vi "TL27_Get_Single_Fault_Snapshot.vi"(0 "GEA2 Reference In":refnum<k24>, 5 "Standalone?":bool, 7 "Snapshot Selection":T2, 11 "Error In":errorcluster) -> (4 "GEA2 Reference Out":refnum<k24>, 6 "Fault Snapshots":T1, 15 "Error Out":errorcluster)   [LabVIEW 2021]
uses:
  subVIs/Snap_Selection.ctl
  D:/Common/LabVIEW GEA2 Toolkit/source/GEA3 DLL Source/GeaCommunication.dll
  Common/LabVIEW GEA2 Toolkit/source/GEA3 DLL Source/GeaCommunication.dll
  subVIs/Snap_Input.ctl
  Common/LabVIEW GEA2 Toolkit/GEA3/type defs/Source_Destination.ctl
  Common/LabVIEW GEA2 Toolkit/GEA3/type defs/ERD Read Data In.ctl
  Common/LabVIEW GEA2 Toolkit/GEA3/library/GEA2_Toolkit.lvlib
panel:
  out "ERD Number":string
  out "ERD Data":string
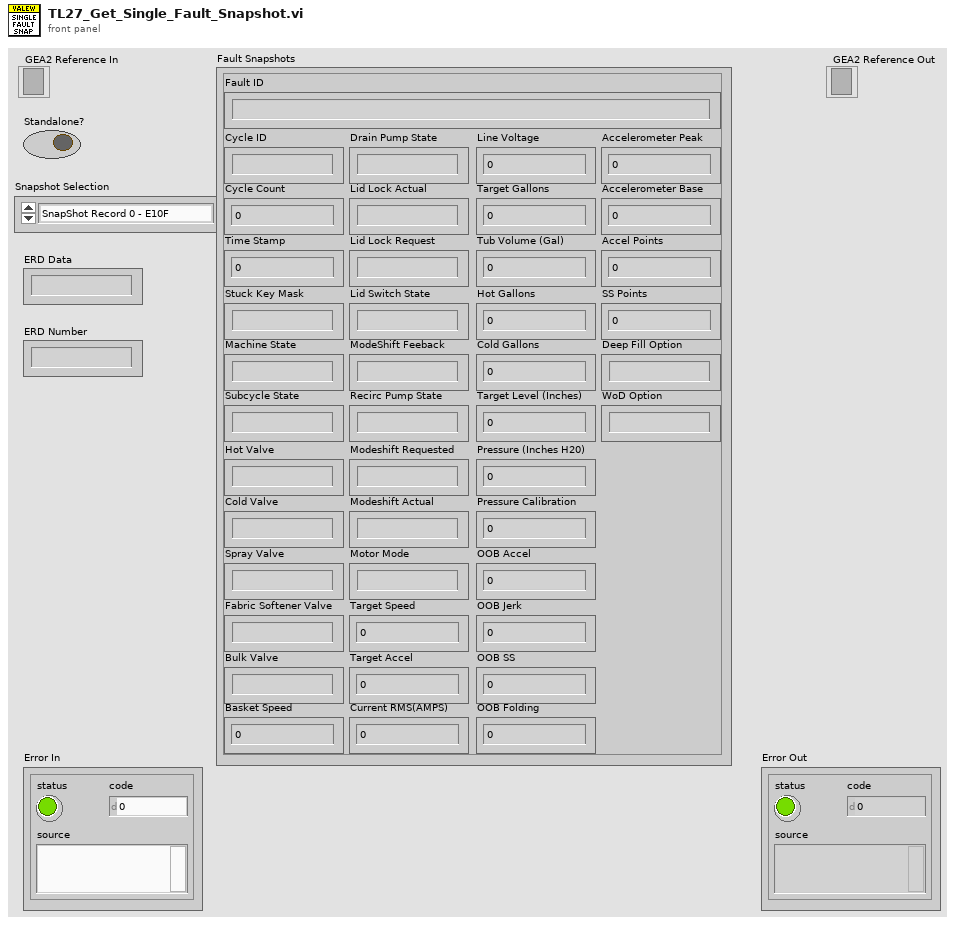
[diagram p1: front panel]
types:
  T1 = typedef "Snap_Input.ctl" = cluster{"Fault ID":string, "Cycle Count":u32, "Cycle ID":string, "Time Stamp":u32, "Stuck Key Mask":string, "Machine State":string, "Subcycle State":string, "Hot Valve":string, "Cold Valve":string, "Spray Valve":string, "Fabric Softener Valve":string, "Bulk Valve":string, "Drain Pump State":string, "Lid Lock Actual":string, "Lid Lock Request":string, "Lid Switch State":string, "ModeShift Feeback":string, "Recirc Pump State":string, "Modeshift Requested":string, "Modeshift Actual":string, "Motor Mode":string, "Target Speed":u16, "Target Accel":u16, "Current RMS(AMPS)":dbl, "Line Voltage":dbl, "Target Gallons":dbl, "Tub Volume (Gal)":dbl, "Hot Gallons":dbl, "Cold Gallons":dbl, "Target Level (Inches)":dbl, "Pressure (Inches H20) ":dbl, "Pressure Calibration":dbl, "OOB Accel":i32, "OOB Jerk":i32, "OOB SS":i32, "OOB Folding":i32, "Accelerometer Peak":i16, "Accelerometer Base":i16, "Accel Points":u8, "SS Points":u8, "Deep Fill Option":string, "WoD Option":string, "Basket Speed":u16}
  T2 = typedef "Snap_Selection.ctl" = enum16{"SnapShot Record 0 - E10F", "Snapshot Record 1 - E110", "Snapshot Record 2 - E111", "Snapshot Record 3 - E112", "Snapshot Record 4 - E113", "Snapshot Record 5 - E114", "Snapshot Record 6 - E115", "Snapshot Record 7 - E116", "Snapshot Record 8 - E117", "Snapshot Record 9 - E118"}
  T3 = typedef "Source_Destination.ctl" = cluster{"Source":u8, "Destination":u8}
  T4 = typedef "ERD Read Data In.ctl" = cluster{"ERD Number":u16, "Data Type":enum16{"string", "boolean", "uint8_t", "uint16_t", "uint32_t", "uint64_t", "int8_t", "int16_t", "int32_t", "int64_t"}}
  T5 = typedef "ERD Read Data Out.ctl" = cluster{"ERD Number":u16, "Data":string}
  T6 = cluster{"ERD Data Out[0]":T5, "ERD Data Out[1]":T5, "ERD Data Out[2]":T5, "ERD Data Out[3]":T5, "ERD Data Out[4]":T5, "ERD Data Out[5]":T5, "ERD Data Out[6]":T5, "ERD Data Out[7]":T5, "ERD Data Out[8]":T5}
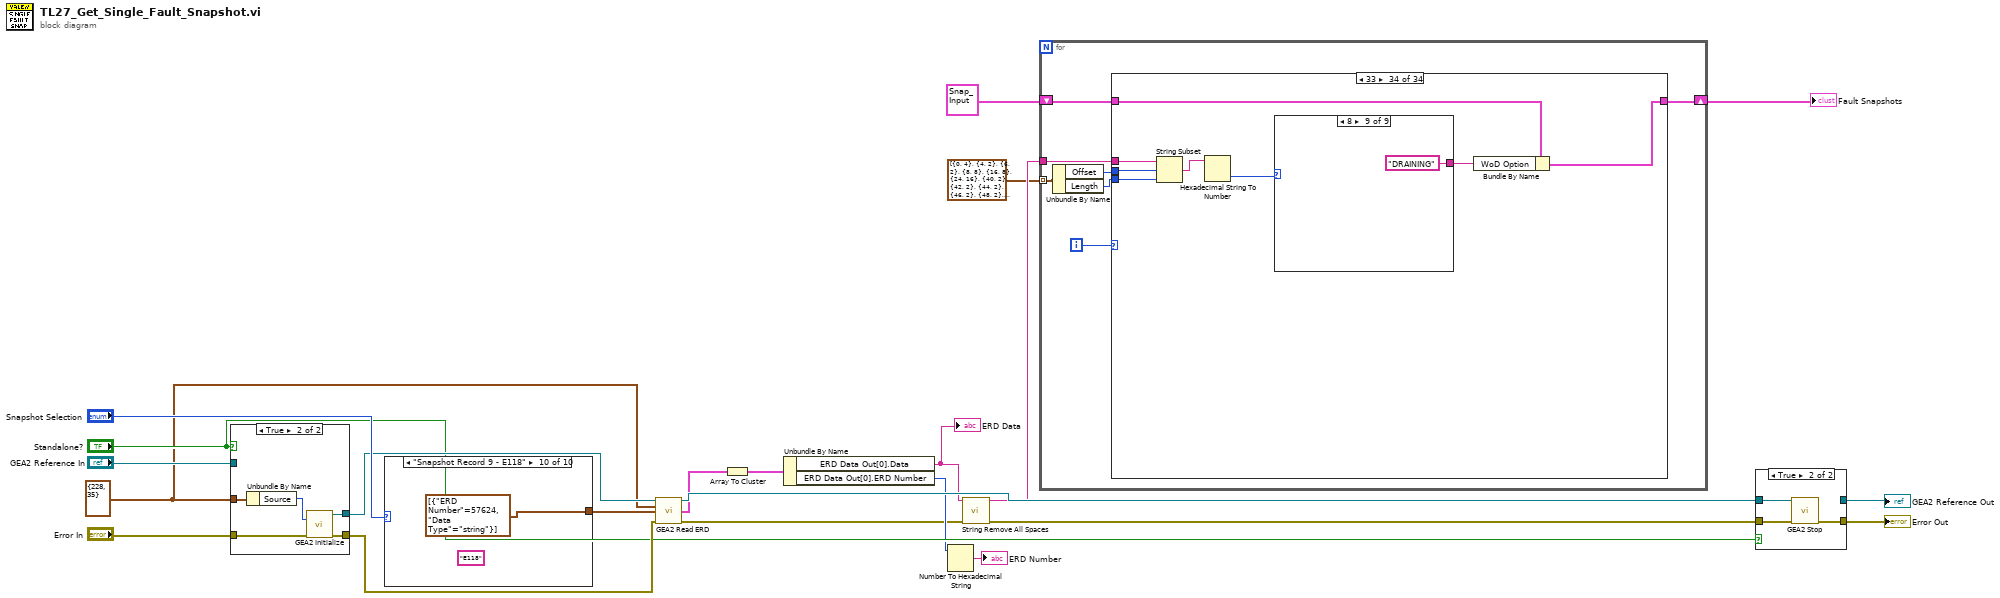
[diagram p0: block diagram]
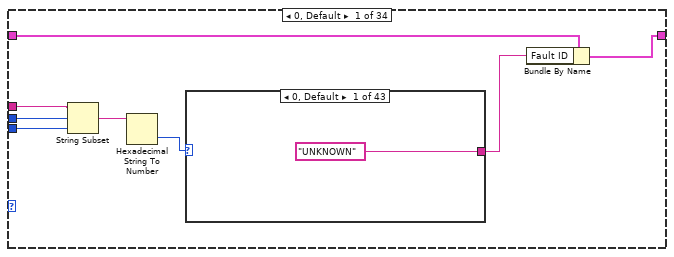
[diagram p2: hidden frame]
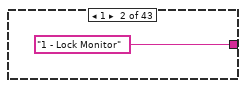
[diagram p3: hidden frame]
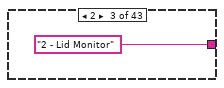
[diagram p4: hidden frame]
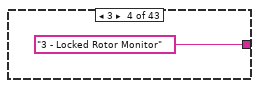
[diagram p5: hidden frame]
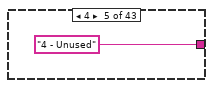
[diagram p6: hidden frame]
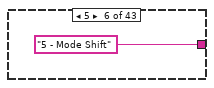
[diagram p7: hidden frame]
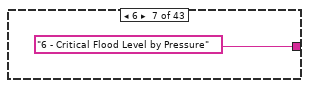
[diagram p8: hidden frame]
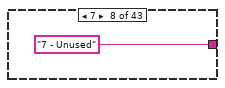
[diagram p9: hidden frame]
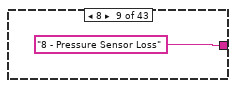
[diagram p10: hidden frame]
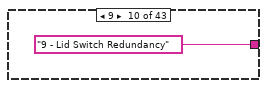
[diagram p11: hidden frame]
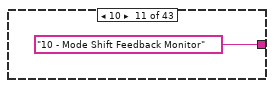
[diagram p12: hidden frame]
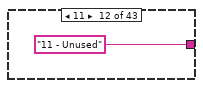
[diagram p13: hidden frame]
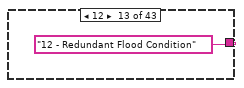
[diagram p14: hidden frame]
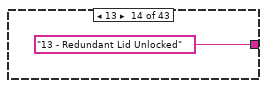
[diagram p15: hidden frame]
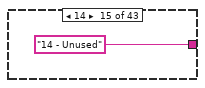
[diagram p16: hidden frame]
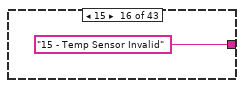
[diagram p17: hidden frame]
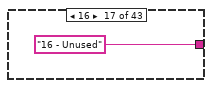
[diagram p18: hidden frame]
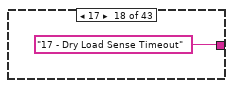
[diagram p19: hidden frame]
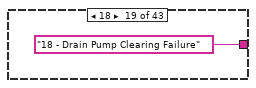
[diagram p20: hidden frame]
diagram:
  w13 = T3 {"Source"=228, "Destination"=35} ("GEA Inputs")
  n1 = case shown="True" "Standalone?" {
    tunnel: "Error In" -> [w23 w29]
    tunnel: [w23 w28] -> w17
    tunnel: "GEA2 Reference In" -> [w24 _]
    tunnel: [w24 w27] -> w18
    tunnel: w13 -> [_ w25]
    frame False {
    }
    frame True {
      n2 = Unbundle By Name(w25) -> ("Source"=w26:u8)
      n3 = call "GEA2 Initialize.vi"("Source Address"=w26, "error in"=w29) -> ("GEA2 Reference Out"=w27:refnum<k24>, "error out"=w28:errorcluster)  [unwired: 10 in, 2 out]
    }
  }
  n4 = case shown="\"Snapshot Record 9 - E118\"" "Snapshot Selection" {
    tunnel: [T4[] [{"ERD Number"=57615, "Data Type"=enum."string"}] ("Read ERD List") T4[] [{"ERD Number"=57616, "Data Type"=enum."string"}] ("Read ERD List") T4[] [{"ERD Number"=57617, "Data Type"=enum."string"}] ("Read ERD List") T4[] [{"ERD Number"=57618, "Data Type"=enum."string"}] ("Read ERD List") T4[] [{"ERD Number"=57619, "Data Type"=enum."string"}] ("Read ERD List") T4[] [{"ERD Number"=57620, "Data Type"=enum."string"}] ("Read ERD List") T4[] [{"ERD Number"=57621, "Data Type"=enum."string"}] ("Read ERD List") T4[] [{"ERD Number"=57622, "Data Type"=enum."string"}] ("Read ERD List") T4[] [{"ERD Number"=57623, "Data Type"=enum."string"}] ("Read ERD List") T4[] [{"ERD Number"=57624, "Data Type"=enum."string"}] ("Read ERD List")] -> w21
    frame "SnapShot Record 0 - E10F", Default {
      (unwired) "E10F"
    }
    frame "Snapshot Record 1 - E110" {
      (unwired) "E110"
    }
    frame "Snapshot Record 2 - E111" {
      (unwired) "E111"
    }
    frame "Snapshot Record 3 - E112" {
      (unwired) "E112"
    }
    frame "Snapshot Record 4 - E113" {
      (unwired) "E113"
    }
    frame "Snapshot Record 5 - E114" {
      (unwired) "E114"
    }
    frame "Snapshot Record 6 - E115" {
      (unwired) "E115"
    }
    frame "Snapshot Record 7 - E116" {
      (unwired) "E116"
    }
    frame "Snapshot Record 8 - E117" {
      (unwired) "E117"
    }
    frame "Snapshot Record 9 - E118" {
      (unwired) "E118"
    }
  }
  n5 = call "GEA2 Read ERD.vi"("GEA2 Reference In"=w18, "GEA Inputs"=w13, "Read ERD List"=w21, "Error In"=w17) -> ("GEA2 Reference Out"=w16:refnum<k24>, "ERD Data Out"=w12:T5[], "Error Out"=w7:errorcluster)  [unwired: 8 in, 1 out]
  n6 = Array To Cluster(array=w12) -> (cluster=w11:T6)
  n7 = Unbundle By Name(w11) -> ("ERD Data Out[0].Data"=w8:string, "ERD Data Out[0].ERD Number"=w10:u16)
  "ERD Data" <- w8
  n8 = Number To Hexadecimal String(2:w10) -> (0:→"ERD Number":string)  [unwired: 1 in]
  n9 = call "String Remove All Spaces.vi"("Input String"=w8, "error in (no error)"=w7) -> ("Spaces Removed"=w4:string, "error out"=w6:errorcluster)  [unwired: 12 in]
  n10 = for {
    tunnel: w4 -> [w46]
    shift-right: [w44] -> w1
    shift-left: T1 {"Fault ID"="", "Cycle Count"=0, "Cycle ID"="", "Time Stamp"=0, "Stuck Key Mask"="", "Machine State"="", "Subcycle State"="", "Hot Valve"="", "Cold Valve"="", "Spray Valve"="", "Fabric Softener Valve"="", "Bulk Valve"="", "Drain Pump State"="", "Lid Lock Actual"="", "Lid Lock Request"="", "Lid Switch State"="", "ModeShift Feeback"="", "Recirc Pump State"="", "Modeshift Requested"="", "Modeshift Actual"="", "Motor Mode"="", "Target Speed"=0, "Target Accel"=0, "Current RMS(AMPS)"=0.0, "Line Voltage"=0.0, "Target Gallons"=0.0, "Tub Volume (Gal)"=0.0, "Hot Gallons"=0.0, "Cold Gallons"=0.0, "Target Level (Inches)"=0.0, "Pressure (Inches H20) "=0.0, "Pressure Calibration"=0.0, "OOB Accel"=0, "OOB Jerk"=0, "OOB SS"=0, "OOB Folding"=0, "Accelerometer Peak"=0, "Accelerometer Base"=0, "Accel Points"=0, "SS Points"=0, "Deep Fill Option"="", "WoD Option"="", "Basket Speed"=0} ("input cluster") -> [w45]
    tunnel: cluster{"Offset":i32, "Length":i32}[] [{"Offset"=0, "Length"=4}, {"Offset"=4, "Length"=2}, {"Offset"=6, "Length"=2}, {"Offset"=8, "Length"=8}, {"Offset"=16, "Length"=8}, {"Offset"=24, "Length"=16}, {"Offset"=40, "Length"=2}, {"Offset"=42, "Length"=2}, {"Offset"=44, "Length"=2}, {"Offset"=46, "Length"=2}, {"Offset"=48, "Length"=2}, {"Offset"=50, "Length"=2}, {"Offset"=52, "Length"=4}, {"Offset"=56, "Length"=4}, {"Offset"=60, "Length"=4}, {"Offset"=64, "Length"=4}, {"Offset"=68, "Length"=4}, {"Offset"=72, "Length"=4}, {"Offset"=76, "Length"=4}, {"Offset"=80, "Length"=4}, {"Offset"=84, "Length"=4}, {"Offset"=88, "Length"=8}, {"Offset"=96, "Length"=8}, {"Offset"=104, "Length"=8}, {"Offset"=112, "Length"=8}, {"Offset"=120, "Length"=8}, {"Offset"=128, "Length"=8}, {"Offset"=136, "Length"=8}, {"Offset"=144, "Length"=4}, {"Offset"=148, "Length"=4}, {"Offset"=152, "Length"=2}, {"Offset"=154, "Length"=2}, {"Offset"=156, "Length"=2}, {"Offset"=158, "Length"=2}] -> [w41] mode=indexing
    i -> [w43]
    n11 = Unbundle By Name(w41) -> ("Offset"=w42:i32, "Length"=w40:i32)
    n12 = case shown="33" w43 {
      tunnel: w46 -> [w53 w105 _ w150 w159 w165 w188 w208 w235 w271 w294 w307 w322 w330 w338 w348 w358 w368 w378 w388 w398 w408 w418 w428 w436 w444 w452 w460 w468 w476 w484 w492 w502 w511]
      tunnel: w42 -> [w52 w104 _ w149 w158 w164 w187 w207 w234 w270 w293 w306 w321 w329 w337 w347 w357 w367 w377 w387 w397 w407 w417 w427 w435 w443 w451 w459 w467 w475 w483 w491 w501 w510]
      tunnel: w40 -> [w51 w103 _ w148 w157 w163 w186 w206 w233 w269 w292 w305 w320 w328 w336 w346 w356 w366 w376 w386 w396 w406 w416 w426 w434 w442 w450 w458 w466 w474 w482 w490 w500 w509]
      tunnel: w45 -> [w54 w102 w145 w152 w156 w167 w190 w205 w237 w273 w296 w309 w324 w332 w340 w350 w360 w370 w380 w390 w400 w410 w420 w430 w438 w446 w454 w462 w470 w478 w486 w494 w499 w513]
      tunnel: [w50 w101 w145 w151 w155 w166 w189 w204 w236 w272 w295 w308 w323 w331 w339 w349 w359 w369 w379 w389 w399 w409 w419 w429 w437 w445 w453 w461 w469 w477 w485 w493 w498 w512] -> w44
      frame 0, Default {
        n13 = String Subset(string=w53, offset (0)=w52, length (rest)=w51) -> (substring=w49:string)
        n14 = Hexadecimal String To Number(string=w49) -> (number=w48:u32)  [unwired: 2 in, 1 out]
        n15 = case shown="0, Default" w48 {
          tunnel: ["UNKNOWN" "1 - Lock Monitor" "2 - Lid Monitor" "3 - Locked Rotor Monitor" "4 - Unused" "5 - Mode Shift" "6 - Critical Flood Level by Pressure" "7 - Unused" "8 - Pressure Sensor Loss" "9 - Lid Switch Redundancy" "10 - Mode Shift Feedback Monitor" "11 - Unused" "12 - Redundant Flood Condition" "13 - Redundant Lid Unlocked" "14 - Unused" "15 - Temp Sensor Invalid" "16 - Unused" "17 - Dry Load Sense Timeout" "18 - Drain Pump Clearing Failure" "19 - UI State Timeout" "20 - Critical Flood Level by Gallons" "21 - Unused " "22 - OOB during dry load sense" "23 - Critical Lid Lock Failure: Can't Lock" "24 - Lid Logic Failure" "25 - Pressure Sensor Dropout" "26 - OOB Redistribution" "27 - Water Accessibility" "28 - ADC Knob Feedback Invalid" "29 - Suds Lock Abatement Failure" "30 - Stuck Button Fault" "31 - OOB Fallback In Final Spin" "32 - Critical Lid Lock Failure: Can't Unlock" "100 - Accelerometer Communication Error" "101 - Max Fill Pressure" "102 - Clock Monitor" "103 - LidLock Failure" "104 - Adaptive Drain" "105 - Max Fill Volume" "106 - Target Spin Speed Timeout" "107 - Target Spin Speed Dropout" "108 - UI-MC Heartbeat Communication Failure" "109 - Event Sequence Buffer Overrun"] -> w47
          frame 0, Default {
          }
          frame 1 {
          }
          frame 2 {
          }
          frame 3 {
          }
          frame 4 {
          }
          frame 5 {
          }
          frame 6 {
          }
          frame 7 {
          }
          frame 8 {
          }
          frame 9 {
          }
          frame 10 {
          }
          frame 11 {
          }
          frame 12 {
          }
          frame 13 {
          }
          frame 14 {
          }
          frame 15 {
          }
          frame 16 {
          }
          frame 17 {
          }
          frame 18 {
          }
          frame 19 {
          }
          frame 20 {
          }
          frame 21 {
          }
          frame 22 {
          }
          frame 23 {
          }
          frame 24 {
          }
          frame 25 {
          }
          frame 26 {
          }
          frame 27 {
          }
          frame 28 {
          }
          frame 29 {
          }
          frame 30 {
          }
          frame 31 {
          }
          frame 32 {
          }
          frame 100 {
          }
          frame 101 {
          }
          frame 102 {
          }
          frame 103 {
          }
          frame 104 {
          }
          frame 105 {
          }
          frame 106 {
          }
          frame 107 {
          }
          frame 108 {
          }
          frame 109 {
          }
        }
        n16 = Bundle By Name(cluster=w54, "Fault ID"=w47) -> (w50:T1)
      }
      frame 1 {
        n17 = String Subset(string=w105, offset (0)=w104, length (rest)=w103) -> (substring=w100:string)
        n18 = Hexadecimal String To Number(string=w100) -> (number=w99:u32)  [unwired: 2 in, 1 out]
        n19 = case shown="0, Default" w99 {
          tunnel: ["0 - NotDefined" "1 - BasketClean" "2 - DrainAndSpin" "3 - QuickRinse" "4 - BulkyItems" "5 - Sanitize" "6 - TowelsSheets" "8 - Normal_Mixedload" "9 - Whites" "10 - DarkColors" "11 - Jeans" "12 - HandWash" "13 - Delicates" "14 - SpeedWash" "15 - HeavyDuty" "16 - Allergen" "17 - PowerClean" "18 - RinseSpin" "19 - SingleItemWash" "20 - Colors" "21 - ColdWash" "22 - WaterOnDemand" "23 - NotUsed_Start" "127 - NotUsed_End" "128 - Cottons" "129 - EasyCare" "130 - ActiveWear" "131 - TimedDry" "132 - DeWrinkle" "133 - QuickAirFluff" "134 - SteamRefresh" "135 - SteamDewrinkle" "136 - SpeedDry" "137 - Mixed" "138 - Quickdry" "139 - Casuals" "140 - Warmup" "141 - EnergySaver" "142 - Antibacterial"] -> w98
          frame 0, Default {
          }
          frame 1 {
          }
          frame 2 {
          }
          frame 3 {
          }
          frame 4 {
          }
          frame 5 {
          }
          frame 6 {
          }
          frame 8 {
          }
          frame 9 {
          }
          frame 10 {
          }
          frame 11 {
          }
          frame 12 {
          }
          frame 13 {
          }
          frame 14 {
          }
          frame 15 {
          }
          frame 16 {
          }
          frame 17 {
          }
          frame 18 {
          }
          frame 19 {
          }
          frame 20 {
          }
          frame 21 {
          }
          frame 22 {
          }
          frame 23 {
          }
          frame 127 {
          }
          frame 128 {
          }
          frame 129 {
          }
          frame 130 {
          }
          frame 131 {
          }
          frame 132 {
          }
          frame 133 {
          }
          frame 134 {
          }
          frame 135 {
          }
          frame 136 {
          }
          frame 137 {
          }
          frame 138 {
          }
          frame 139 {
          }
          frame 140 {
          }
          frame 141 {
          }
          frame 142 {
          }
        }
        n20 = Bundle By Name(cluster=w102, "Cycle ID"=w98) -> (w101:T1)
      }
      frame 2 {
        # "Paddding"
      }
      frame 3 {
        n21 = String Subset(string=w150, offset (0)=w149, length (rest)=w148) -> (substring=w147:string)
        n22 = Hexadecimal String To Number(string=w147) -> (number=w146:u32)  [unwired: 2 in, 1 out]
        n23 = Bundle By Name(cluster=w152, "Cycle Count"=w146) -> (w151:T1)
      }
      frame 4 {
        n24 = String Subset(string=w159, offset (0)=w158, length (rest)=w157) -> (substring=w154:string)
        n25 = Hexadecimal String To Number(string=w154) -> (number=w153:u32)  [unwired: 2 in, 1 out]
        n26 = Bundle By Name(cluster=w156, "Time Stamp"=w153) -> (w155:T1)
      }
      frame 5 {
        (unwired) ""
        n27 = String Subset(string=w165, offset (0)=w164, length (rest)=w163) -> (substring=w162:string)
        n28 = Hexadecimal String To Number(string=w162) -> (number=w161:u32)  [unwired: 2 in, 1 out]
        n29 = case shown="0, Default" w161 {
          tunnel: ["No Stuck Key" "Smart Dispense" "Delay Wash" "Extra Rinse" "Mycycle" "Spin Button" "Deep Rinse" "Soil Button" "Auto Soak" "Temp Button" "Warm Rinse" "Deep Fill" "Water on Demand" "Power Button" "Start Button"] -> w160
          frame 0, Default {
          }
          frame 1 {
          }
          frame 2 {
          }
          frame 4 {
          }
          frame 8 {
          }
          frame 16 {
          }
          frame 32 {
          }
          frame 64 {
          }
          frame 128 {
          }
          frame 256 {
          }
          frame 512 {
          }
          frame 1024 {
          }
          frame 2048 {
          }
          frame 4096 {
          }
          frame 8192 {
          }
        }
        n30 = Bundle By Name(cluster=w167, "Stuck Key Mask"=w160) -> (w166:T1)
      }
      frame 6 {
        n31 = String Subset(string=w188, offset (0)=w187, length (rest)=w186) -> (substring=w185:string)
        n32 = Hexadecimal String To Number(string=w185) -> (number=w184:u32)  [unwired: 2 in, 1 out]
        n33 = case shown="6" w184 {
          tunnel: ["IDLE" "STANDBY" "RUN" "PAUSE" "EOC" "DSM DELAY RUN" "DELAY RUN" "DELAY PAUSE" "DRAIN TIMEOUT" "CLEAN SPEAK"] -> w183
          frame 0, Default {
          }
          frame 1 {
          }
          frame 2 {
          }
          frame 3 {
          }
          frame 4 {
          }
          frame 5 {
          }
          frame 6 {
          }
          frame 7 {
          }
          frame 8 {
          }
          frame 128 {
          }
        }
        n34 = Bundle By Name(cluster=w190, "Machine State"=w183) -> (w189:T1)
      }
      frame 7 {
        n35 = String Subset(string=w208, offset (0)=w207, length (rest)=w206) -> (substring=w203:string)
        n36 = Hexadecimal String To Number(string=w203) -> (number=w202:u32)  [unwired: 2 in, 1 out]
        n37 = case shown="5" w202 {
          tunnel: ["NONE" "FILL" "SOAK" "WASH" "RINSE" "SPIN" "DRAIN" "EXTRA SPIN" "EXTRA RINSE" "TUMBLE" "LOAD SIZE"] -> w201
          frame 0, Default {
          }
          frame 1 {
          }
          frame 2 {
          }
          frame 3 {
          }
          frame 4 {
          }
          frame 5 {
          }
          frame 6 {
          }
          frame 7 {
          }
          frame 8 {
          }
          frame 9 {
          }
          frame 10 {
          }
        }
        n38 = Bundle By Name(cluster=w205, "Subcycle State"=w201) -> (w204:T1)
      }
      frame 8 {
        n39 = String Subset(string=w235, offset (0)=w234, length (rest)=w233) -> (substring=w231:string)
        n40 = Hexadecimal String To Number(string=w231) -> (number=w232:u32)  [unwired: 2 in, 1 out]
        n41 = Number To Boolean Array(number=w232) -> (Boolean array=w230:bool[])
        n42 = Index Array(array=w230) -> (element #1=w229:bool, element #2=w227:bool, element #3=w226:bool, element #4=w225:bool, element #5=w224:bool)  [unwired: 5 in]
        n43 = case shown="False" w229 {
          tunnel: ["OFF" "ON"] -> w228
          frame False {
          }
          frame True {
          }
        }
        n44 = case shown="False" w227 {
          tunnel: ["OFF" "ON"] -> w223
          frame False {
          }
          frame True {
          }
        }
        n45 = case shown="False" w226 {
          tunnel: ["OFF" "ON"] -> w222
          frame False {
          }
          frame True {
          }
        }
        n46 = case shown="False" w225 {
          tunnel: ["OFF" "ON"] -> w221
          frame False {
          }
          frame True {
          }
        }
        n47 = case shown="False" w224 {
          tunnel: ["OFF" "ON"] -> w220
          frame False {
          }
          frame True {
          }
        }
        n48 = Bundle By Name(cluster=w237, "Hot Valve"=w228, "Cold Valve"=w223, "Spray Valve"=w222, "Fabric Softener Valve"=w221, "Bulk Valve"=w220) -> (w236:T1)
      }
      frame 9 {
        n49 = String Subset(string=w271, offset (0)=w270, length (rest)=w269) -> (substring=w268:string)
        n50 = Hexadecimal String To Number(string=w268) -> (number=w267:u32)  [unwired: 2 in, 1 out]
        n51 = Number To Boolean Array(number=w267) -> (Boolean array=w266:bool[])
        n52 = Index Array(array=w266) -> (element #1=w264:bool, element #2=w263:bool, element #3=w260:bool, element #4=w259:bool, element #5=w256:bool, element #6=w255:bool, element #7=w253:bool, element #8=w252:bool)  [unwired: 8 in]
        n53 = Boolean To (0,1)(Boolean=w253) -> (0, 1=w250:i16)
        n54 = Boolean To (0,1)(Boolean=w252) -> (0, 1=w251:i16)
        n55 = Add(x=w250, y=w251) -> (x+y=w249:i16)
        n56 = case shown="True" w256 {
          tunnel: ["AGITATE" "SPIN"] -> w257
          frame False {
          }
          frame True {
          }
        }
        n57 = case shown="True" w255 {
          tunnel: ["OFF" "ON"] -> w254
          frame False {
          }
          frame True {
          }
        }
        n58 = case shown="True" w264 {
          tunnel: ["OFF" "ON"] -> w265
          frame False {
          }
          frame True {
          }
        }
        n59 = case shown="True" w263 {
          tunnel: ["UNLOCKED" "LOCKED"] -> w262
          frame False {
          }
          frame True {
          }
        }
        n60 = case shown="True" w260 {
          tunnel: ["UNLOCKED" "LOCKED"] -> w261
          frame False {
          }
          frame True {
          }
        }
        n61 = case shown="True" w259 {
          tunnel: ["OPEN" "CLOSED"] -> w258
          frame False {
          }
          frame True {
          }
        }
        n62 = case shown="2" w249 {
          tunnel: ["UNKNOWN" "AGITATE" "SPIN"] -> w248
          frame 0, Default {
          }
          frame 1 {
          }
          frame 2 {
          }
        }
        n63 = Bundle By Name(cluster=w273, "Drain Pump State"=w265, "Lid Lock Actual"=w262, "Lid Lock Request"=w261, "Lid Switch State"=w258, "ModeShift Feeback"=w257, "Recirc Pump State"=w254, "Modeshift Requested"=w248) -> (w272:T1)
      }
      frame 10 {
        n64 = String Subset(string=w294, offset (0)=w293, length (rest)=w292) -> (substring=w291:string)
        n65 = Hexadecimal String To Number(string=w291) -> (number=w290:u32)  [unwired: 2 in, 1 out]
        n66 = case shown="4" w290 {
          tunnel: ["UNKNOWN" "AGITATE" "SPIN" "TRANS TO SPIN" "TRANS TO AGITATE"] -> w289
          frame 0, Default {
          }
          frame 1 {
          }
          frame 2 {
          }
          frame 3 {
          }
          frame 4 {
          }
        }
        n67 = Bundle By Name(cluster=w296, "Modeshift Actual"=w289) -> (w295:T1)
      }
      frame 11 {
        n68 = String Subset(string=w307, offset (0)=w306, length (rest)=w305) -> (substring=w304:string)
        n69 = Hexadecimal String To Number(string=w304) -> (number=w303:u32)  [unwired: 2 in, 1 out]
        n70 = case shown="0, Default" w303 {
          tunnel: ["CLOSED LOOP" "CLOSED LOOP ANGLE" "OPEN LOOP" "OPEN LOOP ANGLE" "COASTING" "BRAKING" "IDLE"] -> w302
          frame 0, Default {
          }
          frame 1 {
          }
          frame 2 {
          }
          frame 3 {
          }
          frame 4 {
          }
          frame 5 {
          }
          frame 6 {
          }
        }
        n71 = Bundle By Name(cluster=w309, "Motor Mode"=w302) -> (w308:T1)
      }
      frame 12 {
        n72 = String Subset(string=w322, offset (0)=w321, length (rest)=w320) -> (substring=w319:string)
        n73 = Hexadecimal String To Number(string=w319) -> (number=w318:u32)  [unwired: 2 in, 1 out]
        n74 = To Unsigned Word Integer(number=w318) -> (unsigned 16bit integer=w317:u16)
        n75 = Bundle By Name(cluster=w324, "Target Speed"=w317) -> (w323:T1)
      }
      frame 13 {
        n76 = String Subset(string=w330, offset (0)=w329, length (rest)=w328) -> (substring=w327:string)
        n77 = Hexadecimal String To Number(string=w327) -> (number=w326:u32)  [unwired: 2 in, 1 out]
        n78 = To Unsigned Word Integer(number=w326) -> (unsigned 16bit integer=w325:u16)
        n79 = Bundle By Name(cluster=w332, "Target Accel"=w325) -> (w331:T1)
      }
      frame 14 {
        n80 = String Subset(string=w338, offset (0)=w337, length (rest)=w336) -> (substring=w335:string)
        n81 = Hexadecimal String To Number(string=w335) -> (number=w334:u32)  [unwired: 2 in, 1 out]
        n82 = To Unsigned Word Integer(number=w334) -> (unsigned 16bit integer=w333:u16)
        n83 = Bundle By Name(cluster=w340, "Basket Speed"=w333) -> (w339:T1)
      }
      frame 15 {
        n84 = String Subset(string=w348, offset (0)=w347, length (rest)=w346) -> (substring=w345:string)
        n85 = Hexadecimal String To Number(string=w345) -> (number=w344:u32)  [unwired: 2 in, 1 out]
        n86 = To Double Precision Float(number=w344) -> (double precision float=w343:dbl)
        n87 = Divide(x=w343, y=1024.0) -> (x/y=w341:dbl)
        n88 = Bundle By Name(cluster=w350, "Current RMS(AMPS)"=w341) -> (w349:T1)
      }
      frame 16 {
        n89 = String Subset(string=w358, offset (0)=w357, length (rest)=w356) -> (substring=w355:string)
        n90 = Hexadecimal String To Number(string=w355) -> (number=w354:u32)  [unwired: 2 in, 1 out]
        n91 = To Double Precision Float(number=w354) -> (double precision float=w353:dbl)
        n92 = Divide(x=w353, y=32.0) -> (x/y=w351:dbl)
        n93 = Bundle By Name(cluster=w360, "Line Voltage"=w351) -> (w359:T1)
      }
      frame 17 {
        n94 = String Subset(string=w368, offset (0)=w367, length (rest)=w366) -> (substring=w365:string)
        n95 = Hexadecimal String To Number(string=w365) -> (number=w362:u32)  [unwired: 2 in, 1 out]
        n96 = To Double Precision Float(number=w362) -> (double precision float=w364:dbl)
        n97 = Divide(x=w364, y=100.0) -> (x/y=w361:dbl)
        n98 = Bundle By Name(cluster=w370, "Target Gallons"=w361) -> (w369:T1)
      }
      frame 18 {
        n99 = String Subset(string=w378, offset (0)=w377, length (rest)=w376) -> (substring=w375:string)
        n100 = Hexadecimal String To Number(string=w375) -> (number=w372:u32)  [unwired: 2 in, 1 out]
        n101 = To Double Precision Float(number=w372) -> (double precision float=w374:dbl)
        n102 = Divide(x=w374, y=100.0) -> (x/y=w371:dbl)
        n103 = Bundle By Name(cluster=w380, "Tub Volume (Gal)"=w371) -> (w379:T1)
      }
      frame 19 {
        n104 = String Subset(string=w388, offset (0)=w387, length (rest)=w386) -> (substring=w385:string)
        n105 = Hexadecimal String To Number(string=w385) -> (number=w382:u32)  [unwired: 2 in, 1 out]
        n106 = To Double Precision Float(number=w382) -> (double precision float=w384:dbl)
        n107 = Divide(x=w384, y=100.0) -> (x/y=w381:dbl)
        n108 = Bundle By Name(cluster=w390, "Hot Gallons"=w381) -> (w389:T1)
      }
      frame 20 {
        n109 = String Subset(string=w398, offset (0)=w397, length (rest)=w396) -> (substring=w395:string)
        n110 = Hexadecimal String To Number(string=w395) -> (number=w392:u32)  [unwired: 2 in, 1 out]
        n111 = To Double Precision Float(number=w392) -> (double precision float=w394:dbl)
        n112 = Divide(x=w394, y=100.0) -> (x/y=w391:dbl)
        n113 = Bundle By Name(cluster=w400, "Cold Gallons"=w391) -> (w399:T1)
      }
      frame 21 {
        n114 = String Subset(string=w408, offset (0)=w407, length (rest)=w406) -> (substring=w405:string)
        n115 = Hexadecimal String To Number(string=w405) -> (number=w402:u32)  [unwired: 2 in, 1 out]
        n116 = To Double Precision Float(number=w402) -> (double precision float=w404:dbl)
        n117 = Divide(x=w404, y=1000.0) -> (x/y=w401:dbl)
        n118 = Bundle By Name(cluster=w410, "Target Level (Inches)"=w401) -> (w409:T1)
      }
      frame 22 {
        n119 = String Subset(string=w418, offset (0)=w417, length (rest)=w416) -> (substring=w415:string)
        n120 = Hexadecimal String To Number(string=w415) -> (number=w412:u32)  [unwired: 2 in, 1 out]
        n121 = To Double Precision Float(number=w412) -> (double precision float=w414:dbl)
        n122 = Divide(x=w414, y=1000.0) -> (x/y=w411:dbl)
        n123 = Bundle By Name(cluster=w420, "Pressure (Inches H20)"=w411) -> (w419:T1)
      }
      frame 23 {
        n124 = String Subset(string=w428, offset (0)=w427, length (rest)=w426) -> (substring=w425:string)
        n125 = Hexadecimal String To Number(string=w425) -> (number=w422:u32)  [unwired: 2 in, 1 out]
        n126 = To Double Precision Float(number=w422) -> (double precision float=w424:dbl)
        n127 = Divide(x=w424, y=1000.0) -> (x/y=w421:dbl)
        n128 = Bundle By Name(cluster=w430, "Pressure Calibration"=w421) -> (w429:T1)
      }
      frame 24 {
        n129 = String Subset(string=w436, offset (0)=w435, length (rest)=w434) -> (substring=w433:string)
        n130 = Hexadecimal String To Number(string=w433) -> (number=w431:u32)  [unwired: 2 in, 1 out]
        n131 = To Long Integer(number=w431) -> (32bit integer=w432:i32)
        n132 = Bundle By Name(cluster=w438, "OOB Accel"=w432) -> (w437:T1)
      }
      frame 25 {
        n133 = String Subset(string=w444, offset (0)=w443, length (rest)=w442) -> (substring=w441:string)
        n134 = Hexadecimal String To Number(string=w441) -> (number=w440:u32)  [unwired: 2 in, 1 out]
        n135 = To Long Integer(number=w440) -> (32bit integer=w439:i32)
        n136 = Bundle By Name(cluster=w446, "OOB Jerk"=w439) -> (w445:T1)
      }
      frame 26 {
        n137 = String Subset(string=w452, offset (0)=w451, length (rest)=w450) -> (substring=w449:string)
        n138 = Hexadecimal String To Number(string=w449) -> (number=w447:u32)  [unwired: 2 in, 1 out]
        n139 = To Long Integer(number=w447) -> (32bit integer=w448:i32)
        n140 = Bundle By Name(cluster=w454, "OOB SS"=w448) -> (w453:T1)
      }
      frame 27 {
        n141 = String Subset(string=w460, offset (0)=w459, length (rest)=w458) -> (substring=w457:string)
        n142 = Hexadecimal String To Number(string=w457) -> (number=w455:u32)  [unwired: 2 in, 1 out]
        n143 = To Long Integer(number=w455) -> (32bit integer=w456:i32)
        n144 = Bundle By Name(cluster=w462, "OOB Folding"=w456) -> (w461:T1)
      }
      frame 28 {
        n145 = String Subset(string=w468, offset (0)=w467, length (rest)=w466) -> (substring=w465:string)
        n146 = Hexadecimal String To Number(string=w465) -> (number=w463:u32)  [unwired: 2 in, 1 out]
        n147 = To Word Integer(number=w463) -> (16bit integer=w464:i16)
        n148 = Bundle By Name(cluster=w470, "Accelerometer Peak"=w464) -> (w469:T1)
      }
      frame 29 {
        n149 = String Subset(string=w476, offset (0)=w475, length (rest)=w474) -> (substring=w473:string)
        n150 = Hexadecimal String To Number(string=w473) -> (number=w471:u32)  [unwired: 2 in, 1 out]
        n151 = To Word Integer(number=w471) -> (16bit integer=w472:i16)
        n152 = Bundle By Name(cluster=w478, "Accelerometer Base"=w472) -> (w477:T1)
      }
      frame 30 {
        n153 = String Subset(string=w484, offset (0)=w483, length (rest)=w482) -> (substring=w481:string)
        n154 = Hexadecimal String To Number(string=w481) -> (number=w479:u32)  [unwired: 2 in, 1 out]
        n155 = To Unsigned Byte Integer(number=w479) -> (unsigned 8bit integer=w480:u8)
        n156 = Bundle By Name(cluster=w486, "Accel Points"=w480) -> (w485:T1)
      }
      frame 31 {
        n157 = String Subset(string=w492, offset (0)=w491, length (rest)=w490) -> (substring=w489:string)
        n158 = Hexadecimal String To Number(string=w489) -> (number=w487:u32)  [unwired: 2 in, 1 out]
        n159 = To Unsigned Byte Integer(number=w487) -> (unsigned 8bit integer=w488:u8)
        n160 = Bundle By Name(cluster=w494, "SS Points"=w488) -> (w493:T1)
      }
      frame 32 {
        n161 = String Subset(string=w502, offset (0)=w501, length (rest)=w500) -> (substring=w497:string)
        n162 = Hexadecimal String To Number(string=w497) -> (number=w496:u32)  [unwired: 2 in, 1 out]
        n163 = case shown="2" w496 {
          tunnel: ["OFF" ("Deep Fill Option") "INCREMENTAL FILL" ("Deep Fill Option") "MAX FILL" ("Deep Fill Option")] -> w495
          frame 0, Default {
          }
          frame 1 {
          }
          frame 2 {
          }
        }
        n164 = Bundle By Name(cluster=w499, "Deep Fill Option"=w495) -> (w498:T1)
      }
      frame 33 {
        n165 = String Subset(string=w511, offset (0)=w510, length (rest)=w509) -> (substring=w508:string)
        n166 = Hexadecimal String To Number(string=w508) -> (number=w507:u32)  [unwired: 2 in, 1 out]
        n167 = case shown="8" w507 {
          tunnel: ["IDLE" ("WoD Option") "FILL ACTIVE" ("WoD Option") "FILL PENDING" ("WoD Option") "FILL PAUSED" ("WoD Option") "FILL SOAK" ("WoD Option") "FULL" ("WoD Option") "DISARMED SELECTED" ("WoD Option") "DISARMED DESELECTED" ("WoD Option") "DRAINING" ("WoD Option")] -> w506
          frame 0, Default {
          }
          frame 1 {
          }
          frame 2 {
          }
          frame 3 {
          }
          frame 4 {
          }
          frame 5 {
          }
          frame 6 {
          }
          frame 7 {
          }
          frame 8 {
          }
        }
        n168 = Bundle By Name(cluster=w513, "WoD Option"=w506) -> (w512:T1)
      }
    }
  }
  "Fault Snapshots" <- w1
  n169 = case shown="True" "Standalone?" {
    tunnel: [w523 w527] -> w5
    tunnel: w16 -> [w524 w526]
    tunnel: [w524 _] -> w15
    tunnel: w6 -> [w523 w525]
    frame False {
    }
    frame True {
      n170 = call "GEA2 Stop.vi"("GEA2 Reference In"=w526, "Error In"=w525) -> ("Error Out"=w527:errorcluster)  [unwired: 13 in]
    }
  }
  "GEA2 Reference Out" <- w15
  "Error Out" <- w5
